vi "Configure Dialog.vi"(8 "Error In":errorcluster, 11 "Mute All Msg in":refnum<class "Mute All Msg.lvclass">) -> (0 "Error Out":errorcluster, 2 "OK?":bool, 3 "Mute All Msg out":refnum<class "Mute All Msg.lvclass">)   [LabVIEW 2016, in "KIT-QVA.lvlib" / "Mute All Msg.lvclass"]
doc: "This overrides of this dynamic dispatch VI open the frontpanel to set derived message attributes."
uses:
  Mute All Msg.lvclass
  Mute All Msg.lvclass/Mute All Msg.ctl
panel:
  in  "Mute All":bool
  in  "OK":bool
  in  "Cancel":bool
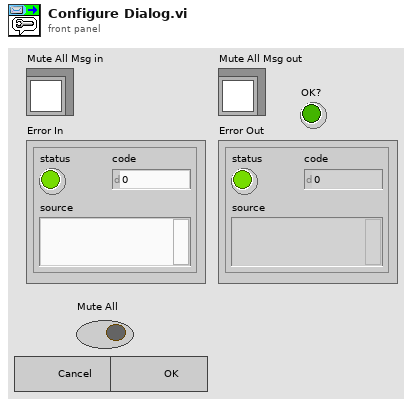
[diagram p1: front panel]
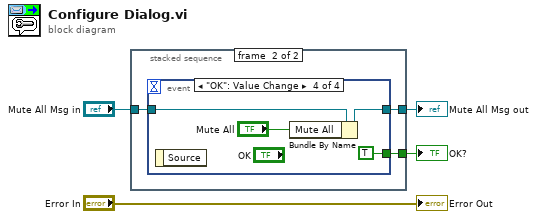
[diagram p0: block diagram]
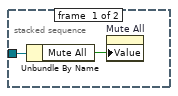
[diagram p2: hidden frame]
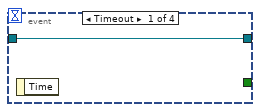
[diagram p3: hidden frame]
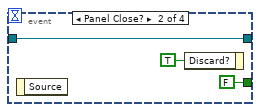
[diagram p4: hidden frame]
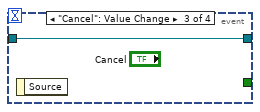
[diagram p5: hidden frame]
diagram:
  n1 = stacked-sequence {
    tunnel: "Mute All Msg in" -> [w6 w9]
    tunnel: [_ w8] -> w2
    tunnel: [_ w7] -> w1
    frame #0 {
      n2 = Unbundle By Name(w6) -> ("Mute All"=w5:bool)
      n3 = property on="Mute All" class="Bool (strict)"("Value"=w5) -> ()  [unwired: 2 in, 2 out]
    }
    frame #1 {
      n4 = event shown="[3] \"OK\": Value Change" {
        selector: _ -> [_ _ _ _]
        dyn-events: _ -> [_ _ _ _]
        timeout: _ -> [_ _ _ _]
        tunnel: [w10 w11 w14 w17] -> w8
        tunnel: w9 -> [w10 w11 w14 w18]
        tunnel: [_ FALSE _ TRUE] -> w7
        event Timeout {
          n5 = event-data() -> ()  [unwired: 1 in, 1 out]
        }
        event Panel Close? {
          n6 = event-data() -> ()  [unwired: 1 in, 1 out]
          n7 = event-data("Discard?"=TRUE) -> ()  [unwired: 1 in, 1 out]
        }
        event "Cancel": Value Change {
          n8 = event-data() -> ()  [unwired: 1 in, 1 out]
        }
        event "OK": Value Change {
          n9 = event-data() -> ()  [unwired: 1 in, 1 out]
          n10 = Bundle By Name(cluster=w18, "Mute All"="Mute All") -> (w17:refnum<class "Mute All Msg.lvclass">)
        }
      }
    }
  }
  "Mute All Msg out" <- w2
  "OK?" <- w1
  "Error Out" <- "Error In"
